vi "Write Parity.vi"(8 "error in (no error)":errorcluster, 10 "parity":u16(ring) items=["None", "Odd", "Even", "Mark", "Space"], 11 "serial slave in":refnum<class "Serial Slave.lvclass">) -> (0 "error out":errorcluster, 3 "serial slave out":refnum<class "Serial Slave.lvclass">)   [LabVIEW 2020, in "SubVIs.lvlib" / "Serial Slave.lvclass"]
uses:
  <vilib>/Modbus/subvis/Protocol/Serial/Serial Slave/Serial Slave.lvclass
  <vilib>/Modbus/subvis/Protocol/Serial/Serial Slave/Serial Slave.lvclass/Serial Slave.ctl
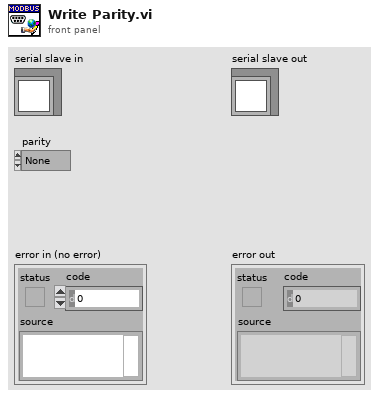
[diagram p1: front panel]
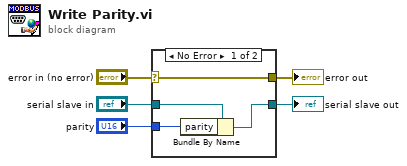
[diagram p0: block diagram]
diagram:
  n1 = case shown="No Error" "error in (no error)" {
    selector: "error in (no error)" -> [w9 w10]
    tunnel: [w9 w10] -> w4
    tunnel: [w7 w11] -> w2
    tunnel: "serial slave in" -> [w8 w11]
    tunnel: "parity" -> [w6 _]
    frame No Error {
      n2 = Bundle By Name(cluster=w8, "parity"=w6) -> (w7:refnum<class "Serial Slave.lvclass">)
    }
    frame Error {
    }
  }
  "error out" <- w4
  "serial slave out" <- w2
